vi "Get Connection String.vi"(4 "Error In":errorcluster, 7 "Config Data_DB_ADO in":refnum<class "Config Data_DB_ADO.lvclass">) -> (0 "Error Out":errorcluster, 2 "Connection String":string, 3 "Config Data_DB_ADO out":refnum<class "Config Data_DB_ADO.lvclass">)   [LabVIEW 2014, in "Config Data.lvlib" / "Config Data_DB_ADO.lvclass"]
uses:
  Config Data_DB_ADO.lvclass
  <vilib>/Utility/config.llb/Read Key (String).vi
  <vilib>/Utility/config.llb/Write Key (String).vi
  <vilib>/Utility/config.llb/NI_LVConfig.lvlib
  Config Data.lvclass
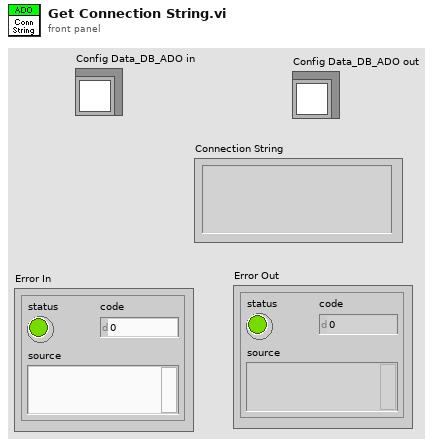
[diagram p1: front panel]
types:
  T1 = typedef "NI_LVConfig.lvlib/Config Data RefNum.ctl" = refnum<k1>
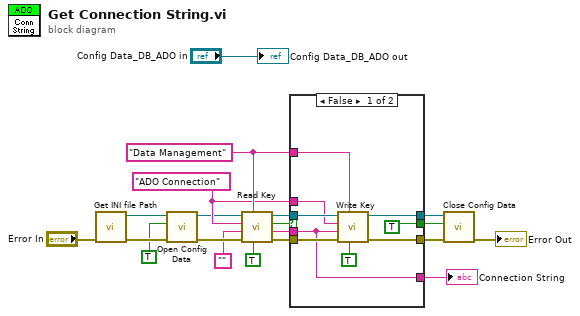
[diagram p0: block diagram]
diagram:
  w16 = "Data Management" ("default value")
  w11 = "ADO Connection" ("default value")
  n1 = call "Get INI file Path.vi"("error in (no error)"="Error In") -> ("error out"=w19:errorcluster, "appended path"=w18:path)  [unwired: 5 in]
  n2 = call <vilib>:"Open Config Data.vi"("error in (no error)"=w19, "create file if necessary (T)"=TRUE ("create file if necessary? (T)"), "configuration file path"=w18) -> ("error out"=w6:errorcluster, "refnum"=w7:T1)  [unwired: 6 in, 1 out]
  n3 = call-poly <vilib>:"Read Key.vi"("read raw string? (F)"=TRUE, "section"=w16, "error in (no error)"=w6, "default value"="", "key"=w11, "refnum"=w7) -> ("error out"=w10:errorcluster, "value"=w12:string, "found?"=w8:bool, "refnum out"=w9:T1)  [unwired: 2 out]
  n4 = case shown="False" w8 {
    tunnel: w9 -> [w28 w31]
    tunnel: w16 -> [w27 _]
    tunnel: w10 -> [w29 w32]
    tunnel: [w24 w32] -> w13
    tunnel: [w25 w31] -> w15
    tunnel: w11 -> [w26 _]
    tunnel: w12 -> [w21 w30]
    tunnel: [TRUE ("write configuration file? (T)") _] -> w14
    tunnel: [w21 w30] -> w1
    frame False {
      n5 = call-poly <vilib>:"Write Key.vi"("write raw string? (F)"=TRUE ("read raw string? (F)"), "section"=w27, "error in (no error)"=w29, "value"=w21, "key"=w26, "refnum"=w28) -> ("error out"=w24:errorcluster, "refnum out"=w25:T1)  [unwired: 4 out]
    }
    frame True {
    }
  }
  "Connection String" <- w1
  n6 = call <vilib>:"Close Config Data.vi"("error in (no error)"=w13, "write file if changed (T)"=w14, "refnum"=w15) -> ("error out"=→"Error Out":errorcluster)  [unwired: 8 out]
  "Config Data_DB_ADO out" <- "Config Data_DB_ADO in"
